vi "Heads or Tails.vi"() -> ()   [LabVIEW 2015]
panel:
  in  "?":bool
  out "new picture 2":picture
  out "new picture":picture
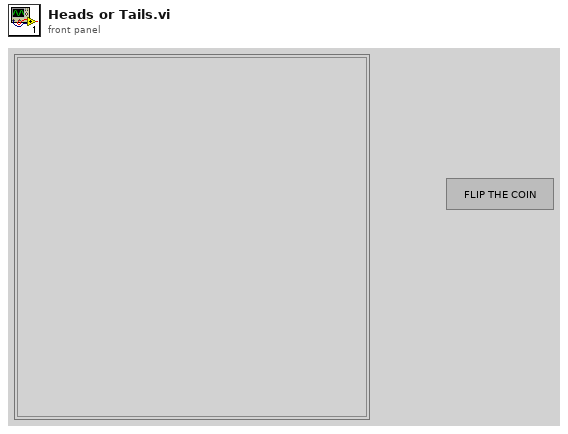
[diagram p1: front panel]
types:
  T1 = typedef "imagedata.ctl" = cluster{"image type":i32, "image depth":i32, "image":u8[], "mask":u8[], "colors":u32[], "Rectangle":cluster{"left":i16, "top":i16, "right":i16, "bottom":i16}}
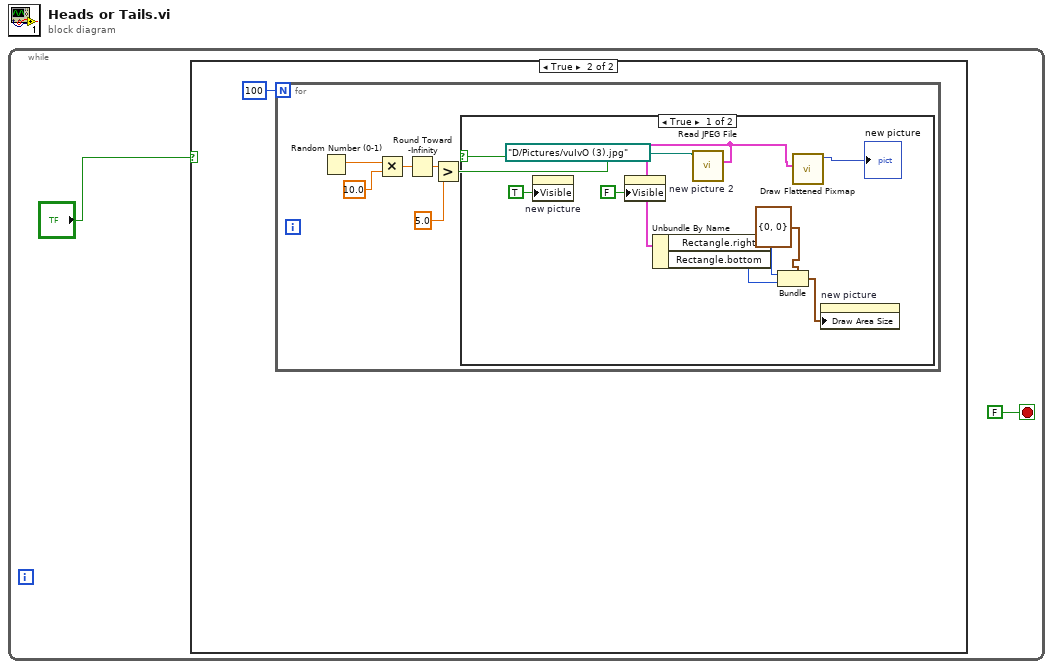
[diagram p0: block diagram]
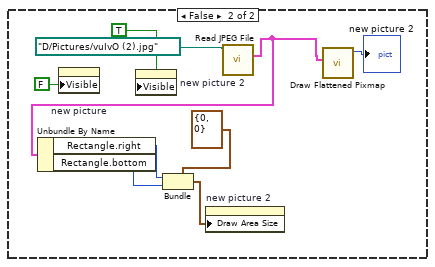
[diagram p3: hidden frame]
diagram:
  n1 = while {
    stop <- FALSE stop-if-true
    n2 = case shown="True" "?" {
      frame False {
      }
      frame True {
        n3 = for {
          N: 100 -> [_]
          n4 = Random Number (0-1)() -> (number: 0 to 1=w9:dbl)
          n5 = Multiply(x=w9, y=10.0) -> (x*y=w7:dbl)
          n6 = Round Toward -Infinity(1:w7) -> (0:w6:dbl)
          n7 = Greater?(x=w6, y=5.0) -> (0:w4:bool)
          n8 = case shown="True" w4 {
            frame True {
              n9 = property on="new picture" class="Pict"("Visible"=TRUE) -> ()  [unwired: 2 in, 2 out]
              n10 = property on="new picture 2" class="Pict"("Visible"=FALSE) -> ()  [unwired: 2 in, 2 out]
              n11 = call <vilib>:"Read JPEG File.vi"("path to JPEG file"=path "D:/Pictures/vuIvO (3).jpg") -> ("image data"=w14:T1)  [unwired: 8 in, 2 out]
              n12 = Unbundle By Name(w14) -> ("Rectangle.right"=w12:i16, "Rectangle.bottom"=w11:i16)
              n13 = Bundle(cluster=cluster{"Width":u32, "Height":u32} {"Width"=0, "Height"=0} ("Draw Area Size"), "Width"=w12, "Height"=w11) -> (w10:cluster{"Width":u32, "Height":u32})
              n14 = call <vilib>:"Draw Flattened Pixmap.vi"("image data"=w14) -> ("new picture"=→"new picture":picture)  [unwired: 8 in]
              n15 = property on="new picture" class="Pict"("Draw Area Size"=w10) -> ()  [unwired: 2 in, 2 out]
            }
            frame False {
              n16 = property on="new picture" class="Pict"("Visible"=FALSE) -> ()  [unwired: 2 in, 2 out]
              n17 = property on="new picture 2" class="Pict"("Visible"=TRUE) -> ()  [unwired: 2 in, 2 out]
              n18 = call <vilib>:"Read JPEG File.vi"("path to JPEG file"=path "D:/Pictures/vuIvO (2).jpg") -> ("image data"=w20:T1)  [unwired: 8 in, 2 out]
              n19 = Unbundle By Name(w20) -> ("Rectangle.right"=w23:i16, "Rectangle.bottom"=w22:i16)
              n20 = Bundle(cluster=cluster{"Height":u32, "Width":u32} {"Height"=0, "Width"=0}, "Height"=w23, "Width"=w22) -> (w21:cluster{"Height":u32, "Width":u32})
              n21 = property on="new picture 2" class="Pict"("Draw Area Size"=w21) -> ()  [unwired: 2 in, 2 out]
              n22 = call <vilib>:"Draw Flattened Pixmap.vi"("image data"=w20) -> ("new picture"=→"new picture 2":picture)  [unwired: 8 in]
            }
          }
        }
      }
    }
  }
